vi "Stop Core.vi"(10 "final error code":i32, 11 "MSS Target Actor in":refnum<class "MSS Target Actor.lvclass">) -> (3 "MSS Target Actor out":refnum<class "MSS Target Actor.lvclass">)   [LabVIEW 2023, in "MSS Target Actor.lvlib" / "MSS Target Actor.lvclass"]
doc: "(<B>Filename</B>: Actor Framework.lvlib:Actor.lvclass:Stop Core.vi)\n\nDefines what the actor does before it stops. Use the <B>final error code</B> input to determine whether the actor shut down in response to an error.\n\nBy default, this method passes the Stop message along to all auto-stop nested actors. A descendant class may override this method to define additional behavior, such as shutting down any processes the actor initiated in its override of the Actor Core method."
uses:
  MSS Target Actor.lvclass
  MSS Target Actor.lvclass/MSS Target Actor.ctl
  <vilib>/ActorFramework/Actor/Actor.lvclass
  Measure and Stimulus Subsystems/Measure and Stimulus Subsystems.lvclass
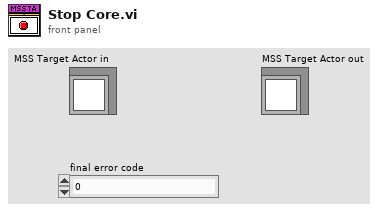
[diagram p1: front panel]
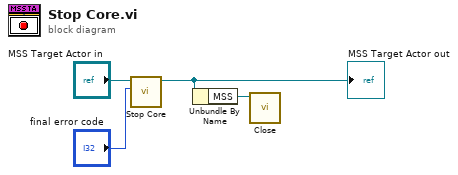
[diagram p0: block diagram]
diagram:
  n1 = call-parent "Stop Core.vi"("final error code"="final error code", "Actor in"="MSS Target Actor in") -> ("Actor out"=w2:refnum<class "MSS Target Actor.lvclass">)  [unwired: 9 in]
  "MSS Target Actor out" <- w2
  n2 = Unbundle By Name(w2) -> ("MSS"=w1:refnum<class "Measure and Stimulus Subsystems.lvclass">)
  n3 = call "Close.vi"("MSS in"=w1) -> ()  [unwired: 9 in, 2 out]
